vi "Set Dialog Position.vi"(4 "error in (no error)":errorcluster, 6 "dialog reference":refnum<vi>, 7 "caller reference":refnum<vi>) -> (0 "error out":errorcluster, 2 "dialog reference out":refnum<vi>, 3 "caller reference out":refnum<vi>)   [LabVIEW 2014]
doc: "This VI calcuates the position of a caller and then centers the dialog's front panel on the caller."
panel:
  # "This VI calcuates the position of a caller and then centers the dialog's front panel on the caller."
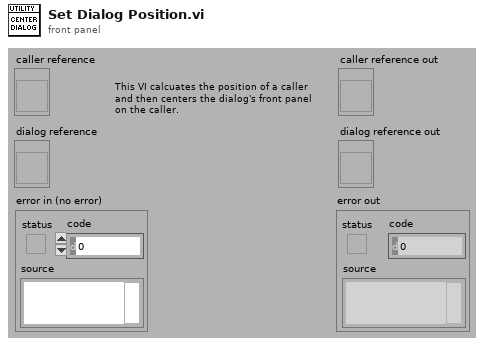
[diagram p1: front panel]
types:
  T1 = enum32{"Invalid", "Standard", "Closed", "Hidden", "Minimized", "Maximized"}
  T2 = typedef "LVRectTypeDef.ctl" = cluster{"Left":i16, "Top":i16, "Right":i16, "Bottom":i16}
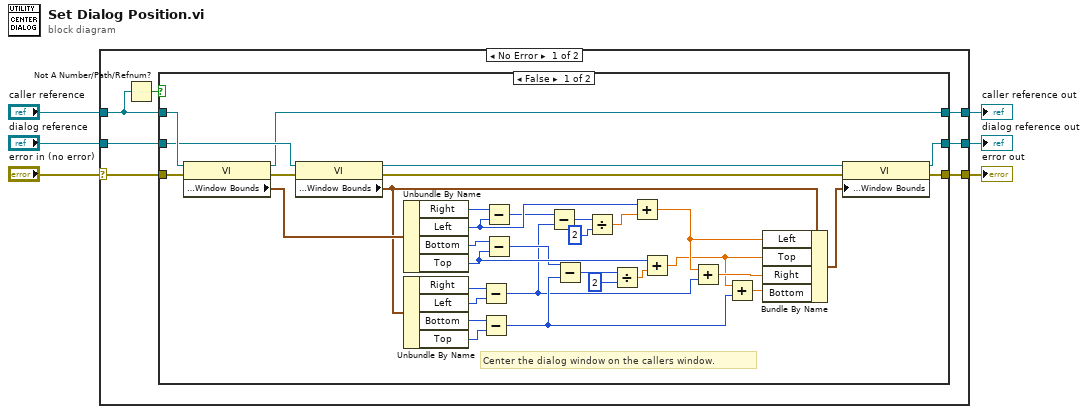
[diagram p0: block diagram]
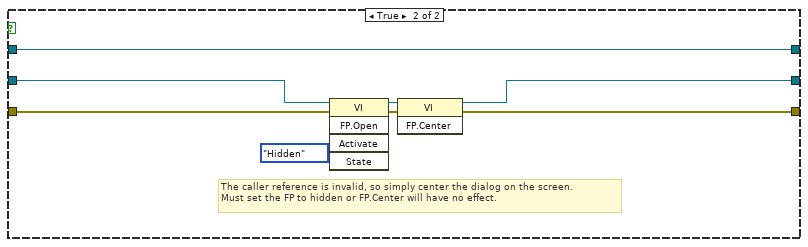
[diagram p2: hidden frame]
diagram:
  n1 = case shown="No Error" "error in (no error)" {
    selector: "error in (no error)" -> [w7 w58]
    tunnel: "dialog reference" -> [w13 w57]
    tunnel: [w12 w56] -> w5
    tunnel: [w11 w57] -> w4
    tunnel: [w10 w58] -> w3
    tunnel: "caller reference" -> [w8 w56]
    frame No Error {
      n2 = Not A Number/Path/Refnum?(number/path/refnum=w8) -> (NaN/Path/Refnum?=w9:bool)
      n3 = case shown="False" w9 {
        tunnel: w8 -> [w47 w53]
        tunnel: w13 -> [w37 w50]
        tunnel: [w35 w53] -> w12
        tunnel: [w34 w54] -> w11
        tunnel: [w33 w55] -> w10
        tunnel: w7 -> [w32 w52]
        frame False {
          # "Center the dialog window on the callers window."
          n4 = property class="VI"(reference=w47, error in=w32) -> (reference out=w35:refnum<vi>, error out=w36:errorcluster, "Front Panel Window:Window Bounds"=w46:T2)
          n5 = property class="VI"(reference=w37, error in=w36) -> (reference out=w40:refnum<vi>, error out=w39:errorcluster, "Front Panel Window:Window Bounds"=w41:T2)
          n6 = Unbundle By Name(w46) -> ("Right"=w28:i16, "Left"=w27:i16, "Bottom"=w26:i16, "Top"=w25:i16)
          n7 = Unbundle By Name(w41) -> ("Right"=w45:i16, "Left"=w44:i16, "Bottom"=w43:i16, "Top"=w42:i16)
          n8 = Subtract(x=w45, y=w44) -> (x-y=w15:i16)
          n9 = Subtract(x=w43, y=w42) -> (x-y=w17:i16)
          n10 = Subtract(x=w28, y=w27) -> (x-y=w16:i16)
          n11 = Subtract(x=w26, y=w25) -> (x-y=w18:i16)
          n12 = Subtract(x=w16, y=w15) -> (x-y=w24:i16)
          n13 = Subtract(x=w18, y=w17) -> (x-y=w21:i16)
          n14 = Divide(x=w24, y=i16 2) -> (x/y=w22:dbl)
          n15 = Divide(x=w21, y=i16 2) -> (x/y=w19:dbl)
          n16 = Add(x=w27, y=w22) -> (x+y=w31:dbl)
          n17 = Add(x=w25, y=w19) -> (x+y=w14:dbl)
          n18 = Add(x=w31, y=w15) -> (x+y=w30:dbl)
          n19 = Add(x=w14, y=w17) -> (x+y=w29:dbl)
          n20 = Bundle By Name(cluster=w41, "Left"=w31, "Top"=w14, "Right"=w30, "Bottom"=w29) -> (w38:T2)
          n21 = property class="VI"(reference=w40, error in=w39, "Front Panel Window:Window Bounds"=w38) -> (reference out=w34:refnum<vi>, error out=w33:errorcluster)
        }
        frame True {
          # "The caller reference is invalid, so simply center the dialog on the screen.\nMust set the FP to hidden or FP.Center will have no effect."
          n22 = invoke class="VI" method="FP.Open"(reference=w50, error in=w52, "State"=T1."Hidden") -> (reference out=w49:refnum<vi>, error out=w51:errorcluster)  [unwired: 2 in, 3 out]
          n23 = invoke class="VI" method="FP.Center"(reference=w49, error in=w51) -> (reference out=w54:refnum<vi>, error out=w55:errorcluster)  [unwired: 1 in, 1 out]
        }
      }
    }
    frame Error {
    }
  }
  "caller reference out" <- w5
  "dialog reference out" <- w4
  "error out" <- w3
